vi "Open Document.vi"(8 "error in (no error)":errorcluster, 11 "File Path":path) -> (0 "error out":errorcluster, 3 "Document out":refnum<class "Document API.lvclass">)   [LabVIEW 2017, in "Document API.lvlib" / "Document API.lvclass"]
doc: "Opens an existing <b>Document out</b> from the <b>Document Path</b> location. Use save to persist your changes.\n\nNotes:\n - If <b>Document Path</b> is empty (default) or is <Not A Path> or is a directory, the VI displays a dialog box from which the user can select a file. Error 43 occurs if you cancel the dialog box. \n - The file extension of the <b>Document Path</b>, or the file selected using the dialog box, is used to determine the file format to create. *.doc or *.docx will create a Word formated document. *.xls or *.xlsx will create an Excel formated document."
uses:
  Document API.lvclass
  Document API.lvclass/Document API.ctl
  NPOI_Document/npoiDocument/npoiDocument.lvclass
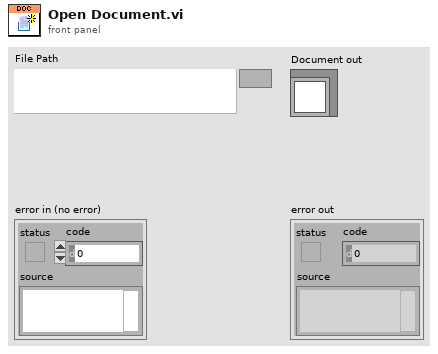
[diagram p1: front panel]
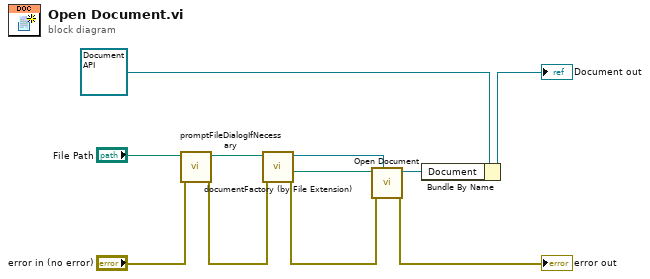
[diagram p0: block diagram]
diagram:
  n1 = call "promptFileDialogIfNecessary.vi"("error in"="error in (no error)", "File Path"="File Path") -> ("error out"=w1:errorcluster, "selected path"=w3:path)  [unwired: 8 in]
  n2 = call "documentFactory (by File Extension).vi"("error in (no error)"=w1, "File Path"=w3) -> ("error out"=w6:errorcluster, "dup file"=w5:path, "npoiDocument out"=w9:refnum<class "npoiDocument.lvclass">)  [unwired: 7 in]
  n3 = call "Open Document.vi"("Document Type"=w9, "error in (no error)"=w6, "Document Path"=w5) -> ("error out"=→"error out":errorcluster, "Document out"=w8:refnum<class "npoiDocument.lvclass">)  [unwired: 7 in]
  n4 = Bundle By Name(cluster=refnum<class "Document API.lvclass"> refnum ("NPOI Document API in"), "Document"=w8) -> (→"Document out":refnum<class "Document API.lvclass">)
